vi "analyse_dosages.vi"(11 "Dosage Cluster":T1(array[cluster])) -> (1 "Cumul Dosages":dbl[](array[numeric]), 2 "Cumul Dos. Times":dbl[](array[numeric]), 3 "Instant. Dos. Times":dbl[](array[numeric]), 4 "Critical Times":dbl[](array[numeric]), 5 "Instant. Dosages":dbl[](array[numeric]), 6 "Critical Dosages":dbl[](array[numeric]), 7 "Total Dosage (kGy)":dbl)   [LabVIEW 2022 SP3]
uses:
  8ab70c4f-4a67-40d2-bc17-1043341c104e.vi
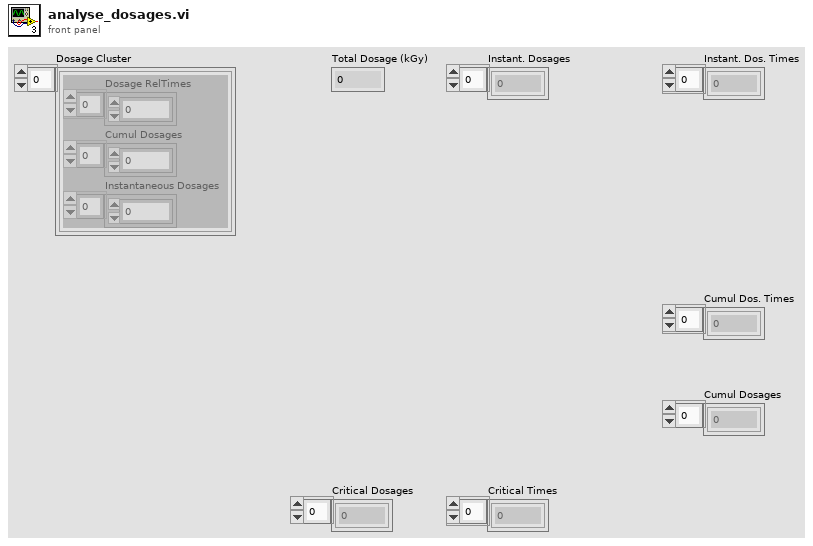
[diagram p1: front panel]
types:
  T1 = cluster{"Dosage RelTimes":dbl[], "Cumul Dosages":dbl[], "Instantaneous Dosages":dbl[]}[]
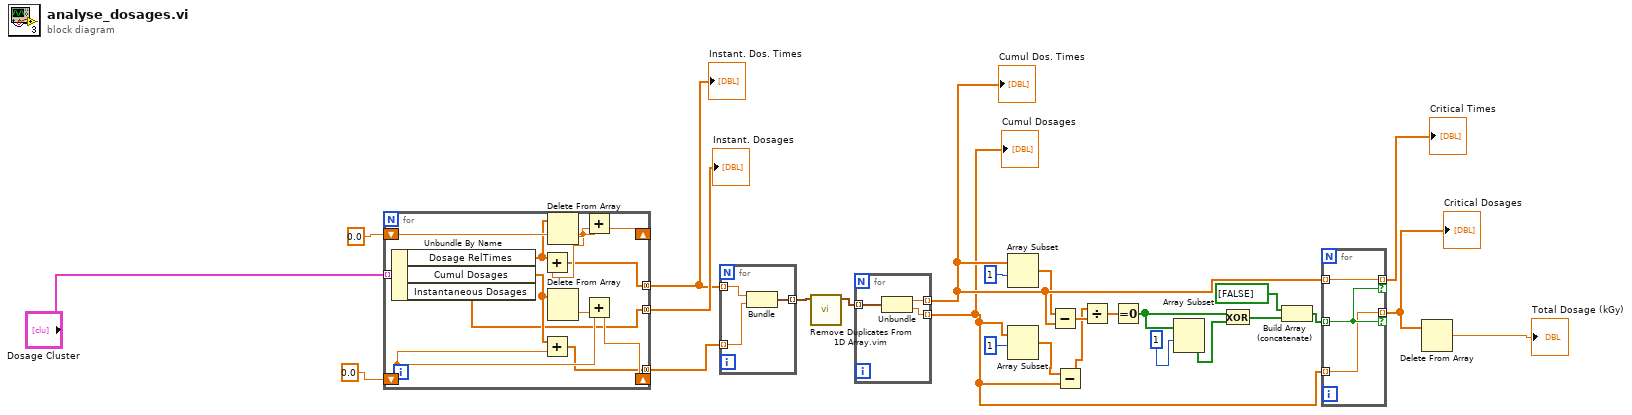
[diagram p0: block diagram]
diagram:
  n1 = for {
    tunnel: "Dosage Cluster" -> [w38] mode=indexing
    tunnel: [w33] -> w24 mode=concatenating
    tunnel: [w28] -> w25 mode=concatenating
    tunnel: [w27] -> w26 mode=concatenating
    shift-right: [w37] -> _
    shift-left: 0.0 -> [w35]
    shift-right: [w30] -> _
    shift-left: 0.0 -> [w31]
    n2 = Unbundle By Name(w38) -> ("Dosage RelTimes"=w34:dbl[], "Cumul Dosages"=w29:dbl[], "Instantaneous Dosages"=w27:dbl[])
    n3 = Add(x=w34, y=w35) -> (x+y=w33:dbl[])
    n4 = Add(x=w29, y=w31) -> (x+y=w28:dbl[])
    n5 = Delete From Array(array=w34) -> (deleted portion=w36:dbl)  [unwired: 2 in, 1 out]
    n6 = Delete From Array(array=w29) -> (deleted portion=w32:dbl)  [unwired: 2 in, 1 out]
    n7 = Add(x=w35, y=w36) -> (x+y=w37:dbl)
    n8 = Add(x=w31, y=w32) -> (x+y=w30:dbl)
  }
  "Instant. Dosages" <- w26
  "Instant. Dos. Times" <- w24
  n9 = for {
    tunnel: w24 -> [w41] mode=indexing
    tunnel: w25 -> [w40] mode=indexing
    tunnel: [w39] -> w15 mode=indexing
    n10 = Bundle(w41, w40) -> (w39:cluster{dbl, dbl})  [unwired: 1 in]
  }
  n11 = call "Remove Duplicates From 1D Array.vim"("array"=w15) -> ("array with duplicates removed"=w16:cluster{dbl, dbl}[])  [unwired: 10 in]
  n12 = for {
    tunnel: w16 -> [w44] mode=indexing
    tunnel: [w43] -> w18 mode=indexing
    tunnel: [w42] -> w17 mode=indexing
    n13 = Unbundle(w44) -> (w43:dbl, w42:dbl)
  }
  "Cumul Dos. Times" <- w18
  "Cumul Dosages" <- w17
  n14 = Array Subset(array=w18, index=1) -> (w2:dbl[])  [unwired: 1 in]
  n15 = Array Subset(array=w17, index=1) -> (w4:dbl[])  [unwired: 1 in]
  n16 = Subtract(x=w2, y=w18) -> (x-y=w10:dbl[])
  n17 = Subtract(x=w4, y=w17) -> (x-y=w9:dbl[])
  n18 = Divide(x=w9, y=w10) -> (x/y=w5:dbl[])
  n19 = Equal To 0?(x=w5) -> (x = 0?=w7:bool[])
  n20 = Array Subset(array=w7, index=1) -> (w8:bool[])  [unwired: 1 in]
  n21 = Exclusive Or(1:w8, 2:w7) -> (0:w12:bool[])
  n22 = Build Array (concatenate)(bool[] [FALSE], w12) -> (w13:bool[])
  n23 = for {
    tunnel: w18 -> [w47] mode=indexing
    tunnel: w13 -> [w46] mode=indexing
    tunnel: [w47] -> w14 mode=indexing if=w46
    tunnel: [w45] -> w19 mode=indexing if=w46
    tunnel: w17 -> [w45] mode=indexing
  }
  "Critical Dosages" <- w19
  "Critical Times" <- w14
  n24 = Delete From Array(array=w19) -> (deleted portion=→"Total Dosage (kGy)":dbl)  [unwired: 2 in, 1 out]
